vi "DAQNavi Read (Analog 1D Wfm NChan NSamp).vi"(8 "error in (no error)":errorcluster, 9 "number of samples per channel to read":u32=1000, 10 "timeout":dbl=10.0 format="%0.2f", 11 "task in":i32) -> (0 "error out":errorcluster, 1 "markBuf":cluster{"DataIndex":i64, "SrcId":i64}[](array[cluster]), 2 "data":waveform(dbl)[](array[waveform]), 3 "task out":i32)   [LabVIEW 2020]
uses:
  DAQNavi_LV.dll
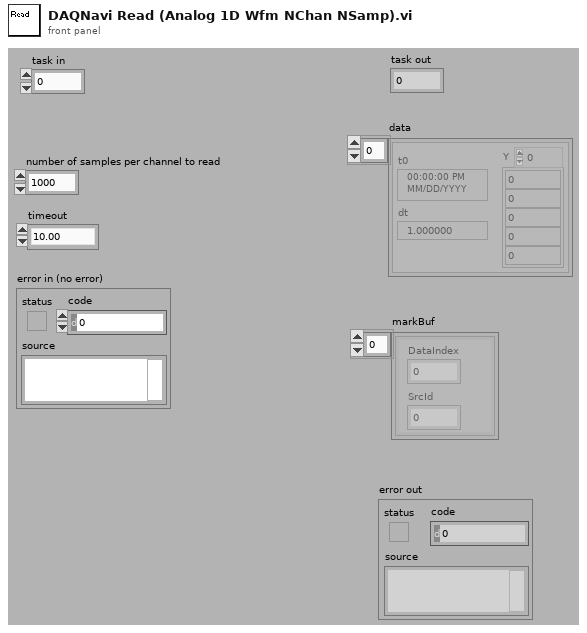
[diagram p1: front panel]
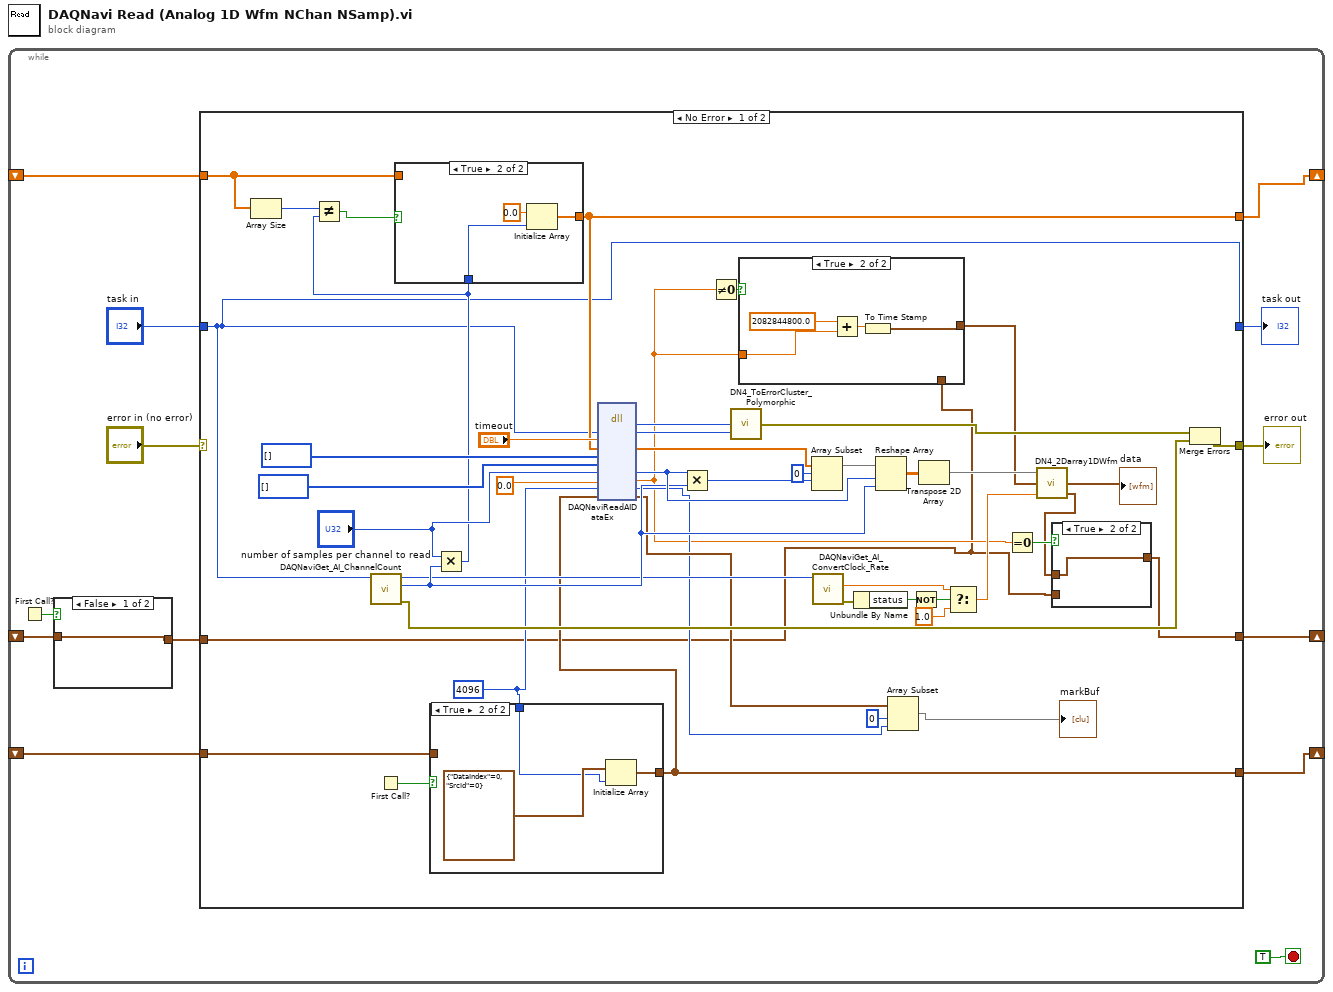
[diagram p0: block diagram]
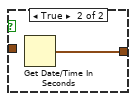
[diagram p2: hidden frame]
diagram:
  n1 = while {
    shift-right: [w5] -> _
    shift-left: _ -> [w7]
    shift-right: [w4] -> _
    shift-left: _ -> [w3]
    shift-right: [w2] -> _
    shift-left: _ -> [w1]
    stop <- TRUE stop-if-true
    n2 = First Call?() -> (First Call?: T/F=w8:bool)
    n3 = case shown="False" w8 {
      tunnel: [w14 w15] -> w6
      tunnel: w7 -> [w14 _]
      frame False {
      }
      frame True {
        n4 = Get Date/Time In Seconds() -> (seconds since 1Jan1904=w15:timestamp)
      }
    }
    n5 = case shown="No Error" "error in (no error)" {
      selector: "error in (no error)" -> [_ w81]
      tunnel: "task in" -> [w20 w82]
      tunnel: [w20 w82] -> w11
      tunnel: [w59 w81] -> w10
      tunnel: w6 -> [w17 w80]
      tunnel: [w34 w80] -> w5
      tunnel: [w29 w79] -> w4
      tunnel: w3 -> [w33 w79]
      tunnel: [w25 w78] -> w2
      tunnel: w1 -> [w26 w78]
      frame No Error {
        w27 = 4096
        n6 = Array Size(array=w33) -> (size(s)=w30:i32)
        n7 = call "DAQNaviGet_AI_ChannelCount.vi"("task in"=w20) -> ("error out"=w49:errorcluster, "channel count"=w50:i32, "task out"=w48:i32)  [unwired: 1 in, 7 out]
        n8 = First Call?() -> (First Call?: T/F=w28:bool)
        n9 = case shown="True" w28 {
          tunnel: [w63 w65] -> w25
          tunnel: w27 -> [_ w64]
          tunnel: w26 -> [w63 _]
          frame False {
          }
          frame True {
            n10 = Initialize Array(cluster{"DataIndex":i64, "SrcId":i64} {"DataIndex"=0, "SrcId"=0}, w64) -> (w65:cluster{"DataIndex":i64, "SrcId":i64}[])
          }
        }
        n11 = Multiply(x="number of samples per channel to read", y=w50) -> (x*y=w31:u32)
        n12 = Not Equal?(x=w30, y=w31) -> (x != y?=w32:bool)
        n13 = case shown="True" w32 {
          tunnel: [w67 w69] -> w29
          tunnel: w31 -> [_ w68]
          tunnel: w33 -> [w67 _]
          frame False {
          }
          frame True {
            n14 = Initialize Array(0.0 ("element"), w68) -> (w69:dbl[])
          }
        }
        n15 = dll-call lib="DAQNavi_LV.dll" fn="DAQNaviReadAIDataEx"("taskID"=w20, "timeout"="timeout", "scaledData"=w29, "rawData16"=u16[] [] ("rawData32"), "rawData32"=u32[] [] ("scaledData"), "samples"="number of samples per channel to read", "startTime"=0.0, "markCount"=w27, "markBuf"=w25) -> ("return type"=w61:i32, "taskID"=w38:i32, "scaledData"=w52:dbl[], "samples"=w55:u32, "startTime"=w18:dbl, "markCount"=w22:i32, "markBuf"=w24:cluster{"DataIndex":i64, "SrcId":i64}[])  [unwired: 4 in, 4 out]
        n16 = Multiply(x=w55, y=w50) -> (x*y=w56:u32)
        n17 = Not Equal To 0?(x=w18) -> (x != 0?=w19:bool)
        n18 = call "DN4_ToErrorCluster_Polymorphic.vi"("task id"=w38, "error code"=w61) -> ("error out"=w58:errorcluster)  [unwired: 3 out]
        n19 = case shown="True" w19 {
          tunnel: w18 -> [_ w77]
          tunnel: [w73 w74] -> w16
          tunnel: w17 -> [w73 _]
          frame False {
          }
          frame True {
            n20 = Add(x=2082844800.0, y=w77) -> (x+y=w75:dbl)
            n21 = To Time Stamp(1:w75) -> (0:w74:timestamp)
          }
        }
        n22 = Array Subset(array=w52, index=0, length=w56) -> (w57:dbl[])
        n23 = call "DAQNaviGet_AI_ConvertClock_Rate.vi"("task in"=w48) -> ("error out"=w47:errorcluster, "rate"=w44:dbl)  [unwired: 1 in, 8 out]
        n24 = Unbundle By Name(w47) -> ("status"=w46:bool)
        n25 = Reshape Array(w57, w55, w50) -> (w51:dbl[][])
        n26 = Array Subset(array=w24, index=0, length=w22) -> (→"markBuf":cluster{"DataIndex":i64, "SrcId":i64}[])
        n27 = Not(x=w46) -> (.not. x?=w45:bool)
        n28 = Transpose 2D Array(2D array=w51) -> (transposed array=w42:dbl[][])
        n29 = Select(t=w44, s=w45, f=1.0) -> (s? t:f=w41:dbl)
        n30 = Equal To 0?(x=w18) -> (x = 0?=w36:bool)
        n31 = call "DN4_2Darray1DWfm.vi"("rate"=w41, "StartTime"=w16, "2D Array"=w42) -> ("EndTime"=w35:timestamp, "1D Wfm"=→"data":waveform(dbl)[])  [unwired: 1 out]
        n32 = case shown="True" w36 {
          tunnel: w35 -> [_ w72]
          tunnel: w17 -> [w71 _]
          tunnel: [w71 w72] -> w34
          frame False {
          }
          frame True {
          }
        }
        n33 = Merge Errors(w58, w49) -> (w59:errorcluster)
      }
      frame Error {
      }
    }
    "task out" <- w11
    "error out" <- w10
  }
